vi "GetTestsFromPackedProjectLibrary.vi"(0 "Packed Project Library Path":path, 11 "error in (no error)":errorcluster) -> (4 "Tests":path[](array[path]), 15 "error out":errorcluster)   [LabVIEW 2016, in "Drona.lvlib"]
uses:
  Drona.lvlib
  <vilib>/Utility/LVLibp/NI_PackedLibraryUtility.lvlib
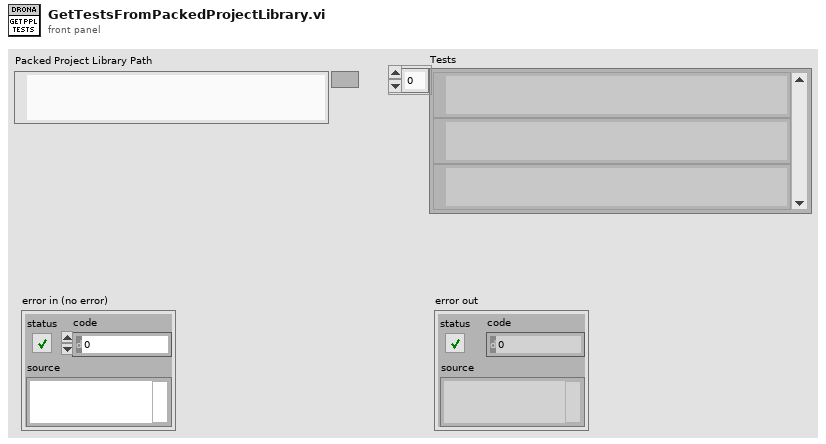
[diagram p1: front panel]
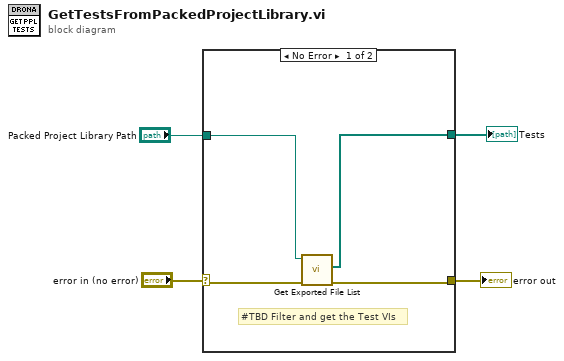
[diagram p0: block diagram]
diagram:
  n1 = case shown="No Error" "error in (no error)" {
    selector: "error in (no error)" -> [w8 w9]
    tunnel: [w5 w9] -> w3
    tunnel: "Packed Project Library Path" -> [w7 _]
    tunnel: [w6 _] -> w1
    frame No Error {
      # "#TBD Filter and get the Test VIs"
      n2 = call <vilib>:"Get Exported File List.vi"("error in (no error)"=w8, "packed library path"=w7) -> ("error out"=w5:errorcluster, "paths"=w6:path[])  [unwired: 7 in, 1 out]
    }
    frame Error {
    }
  }
  "error out" <- w3
  "Tests" <- w1
